vi "CRC.vi"(1 "byte array":u8[](array[numeric]) format="%x") -> (0 "CRCbytes":u8[](array[numeric]), 2 "CRC-CCIT":u16 format="%.0x")   [LabVIEW 2013]
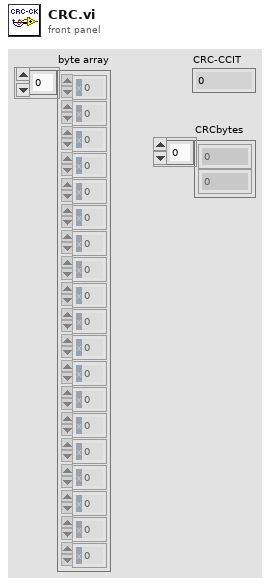
[diagram p1: front panel]
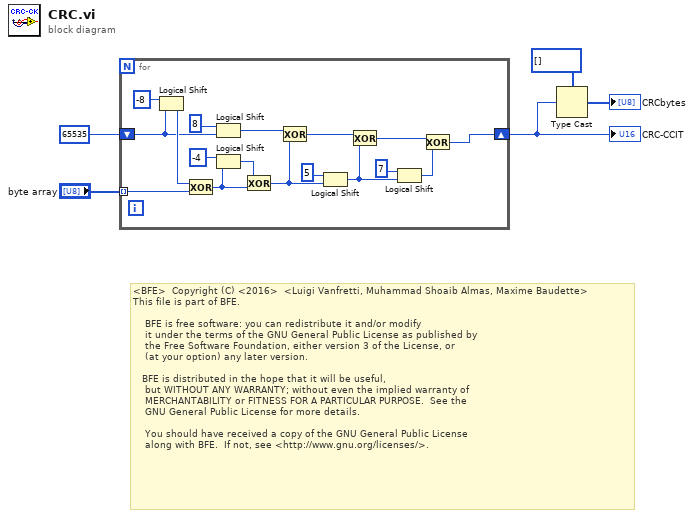
[diagram p0: block diagram]
diagram:
  # "<BFE>  Copyright (C) <2016>  <Luigi Vanfretti, Muhammad Shoaib Almas, Maxime Baudette> \nThis file is part of BFE.\n\n    BFE is free software: you can redistribute it and/or modify\n    it under the terms of the GNU General Public License as published by\n    the Free Software Foundation, either version 3 of the License, or\n    (at your option) any later version.\n\n   BFE is distributed in the hope that it will be useful,\n    but WITHOUT ANY WARRANTY; without even the implied warranty of\n    MERCHANTABILITY or FITNESS FOR A PARTICULAR PURPOSE.  See the\n    GNU General Public License for more details.\n\n    You should have received a copy of the GNU General Public License\n    along with BFE.  If not, see <http://www.gnu.org/licenses/>."
  n1 = for {
    tunnel: "byte array" -> [w20] mode=indexing
    shift-right: [w6] -> w3
    shift-left: u16 65535 -> [w19]
    n2 = Logical Shift(y=i8 -8, x=w19) -> (x << y=w21:u16)
    n3 = Exclusive Or(1:w20, 2:w21) -> (0:w16:u16)
    n4 = Logical Shift(y=i8 8, x=w19) -> (x << y=w14:u16)
    n5 = Logical Shift(y=i8 -4, x=w16) -> (x << y=w15:u16)
    n6 = Exclusive Or(1:w16, 2:w15) -> (0:w13:u16)
    n7 = Exclusive Or(1:w13, 2:w14) -> (0:w11:u16)
    n8 = Logical Shift(y=i8 5, x=w13) -> (x << y=w9:u16)
    n9 = Exclusive Or(1:w9, 2:w11) -> (0:w8:u16)
    n10 = Logical Shift(y=i8 7, x=w9) -> (x << y=w7:u16)
    n11 = Exclusive Or(1:w7, 2:w8) -> (0:w6:u16)
  }
  "CRC-CCIT" <- w3
  n12 = Type Cast(type=u8[] [], x=w3) -> (*(type *) &x=→"CRCbytes":u8[])
